vi "filter.wait.for.command.vi"(11 "filter.data in":T1 {"memory.command"."order.slot.value"."Quantity" format="%016x"; "memory.command"."order.slot.value"."OrderId" format="%016x"; "memory.command"."ticker.slot.value"."Symbol" format="%016x"; "Scratch"."OrderId" format="%016x"}) -> (2 "Ready.for.OrderBook.Command.Input":bool, 3 "filter.data out":T1 {"memory.command"."order.slot.value"."Quantity" format="%016x"; "memory.command"."order.slot.value"."OrderId" format="%016x"; "memory.command"."ticker.slot.value"."Symbol" format="%016x"; "Scratch"."OrderId" format="%016x"})   [LabVIEW 2022 SP3]
uses:
  filter.data.ctl
  filter.states.ctl
  filter.debug.ctl
  filter.debug.slot.ctl
  filter.data.scratch.ctl
  arty/orderbook/orderbook.command.ctl
  arty/orderbook/orderbook.command.type.ctl
  filter.memory.command.ctl
  ticker.slot.ctl
  order.slot.ctl
  <vilib>/rvi/Emulation/niFpgaEmulationIsFPGAContextNoSignature.vi
  <vilib>/rvi/Emulation/niFpgaSctlEmulationGetInTimedLoop.vi
  <vilib>/rvi/errors/niFpgaSetErrorForExecOnDevCompSimple.vi
  <vilib>/rvi/eio/common/nirviEmuReportErrorAndStop.vi
  <vilib>/rvi/DataTransferAndStorage/Container/Common/niFpgaContainerGetUniqueNameForEmu.vi
  <vilib>/rvi/FIFO/Fifo_Resource/nirvififoEmulationSetSize.vi
  <vilib>/rvi/FIFO/Fifo_Resource/nirviFifoEmulationQueueMgr.vi
  <instcachedir>/0/nirviFifoEmulationQueueMgr_E5CAEC123FF24DC58D834DCA3CDAA9B5.lvgen/nirviFifoEmulationQueueMgr_E5CAEC123FF24DC58D834DCA3CDAA9B5_017.vi
  <vilib>/Utility/error.llb/Clear Errors.vi
  <vilib>/rvi/FIFO/Fifo_Resource/nirvififoEmulationCreateLock.vi
  <vilib>/rvi/Emulation/niFpgaProcessEmulError.vi
  <vilib>/rvi/FIFO/Fifo_Resource/nirvififoEmulationObtainLock.vi
  <vilib>/rvi/FIFO/Fifo_Resource/nirvififoEmulationReleaseLock.vi
  <vilib>/rvi/occurrence/nirviWaitOnOccurrenceBase.vi
  <vilib>/rvi/errors/nirviReportUnexpectedCaseInternalError.vi
  <vilib>/rvi/errors/nirviReportUnexpectedCaseInternalError (U32).vi
  <vilib>/rvi/DataTransferAndStorage/Container/XNode/niFpgaContainer.xnode
  <vilib>/rvi/FIFO/Fifo_Resource/nirvififoEmulationRead.vi
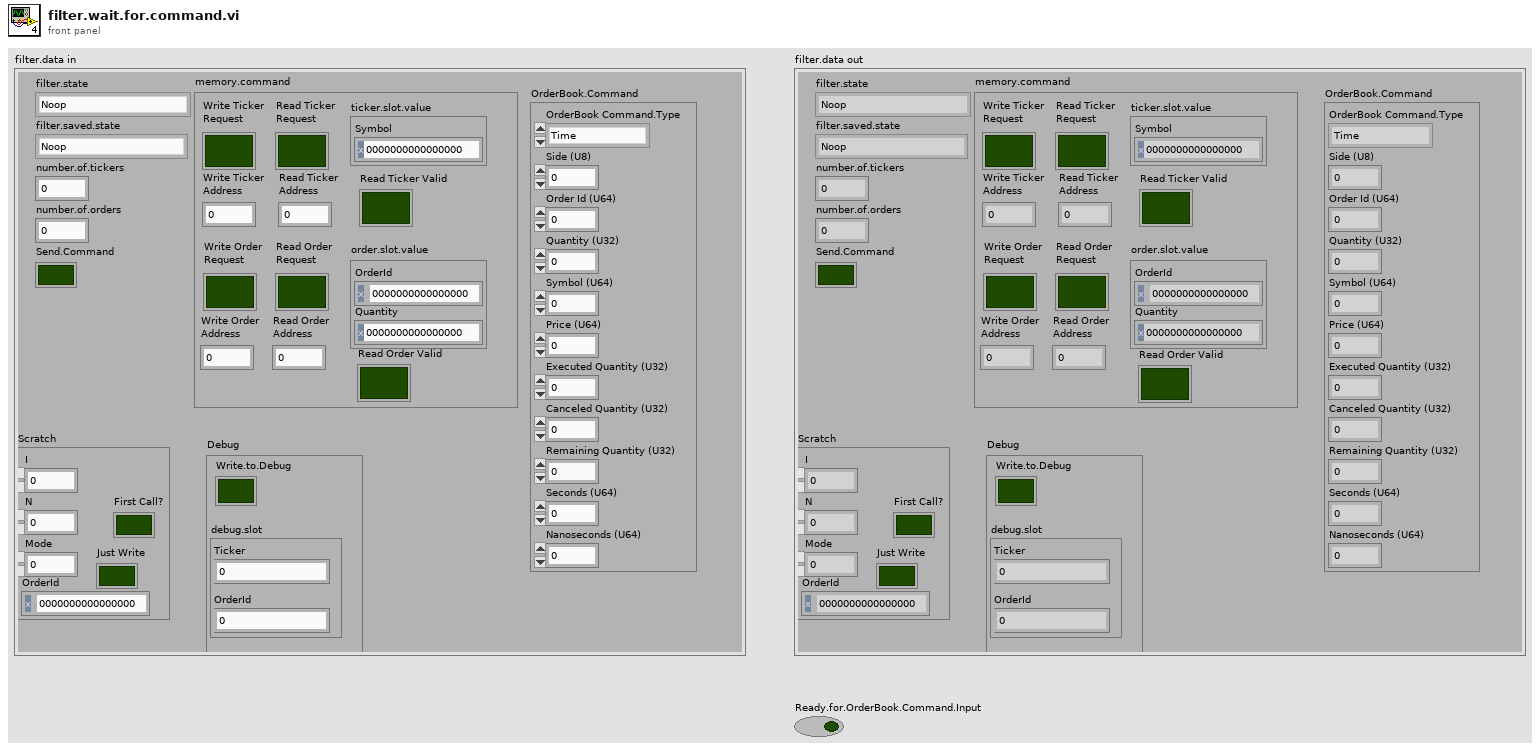
[diagram p1: front panel]
types:
  T1 = typedef "filter.data.ctl" = cluster{"filter.state":T2, "Debug":T3, "number.of.tickers":u32, "number.of.orders":u32, "filter.saved.state":T2, "Scratch":T5, "OrderBook.Command":T6, "Send.Command":bool, "memory.command":T8}
  T2 = typedef "filter.states.ctl" = enum16{"Noop", "Reset", "Debug", "Configuration", "Wait.for.Command", "Filter.Add", "Filter.Other", "Insert.Order", "Delete Order"}
  T3 = typedef "filter.debug.ctl" = cluster{"Write.to.Debug":bool, "debug.slot":T4}
  T4 = typedef "filter.debug.slot.ctl" = cluster{"Ticker":u64, "OrderId":u64}
  T5 = typedef "filter.data.scratch.ctl" = cluster{"I":u32, "N":u32, "Mode":u32, "OrderId":u64, "First Call?":bool, "Just Write":bool}
  T6 = typedef "orderbook.command.ctl" = cluster{"OrderBook Command.Type":T7, "Side (U8)":u8, "Order Id (U64)":u64, "Quantity (U32)":u32, "Symbol (U64)":u64, "Price (U64)":u64, "Executed Quantity (U32)":u32, "Canceled Quantity (U32)":u32, "Remaining Quantity (U32)":u32, "Seconds (U64)":u64, "Nanoseconds (U64)":u64}
  T7 = typedef "orderbook.command.type.ctl" = enum16{"Time", "AddOrder", "OrderExecuted", "OrderExecutedAtPrice", "ReduceSize", "ModifyOrder", "DeleteOrder", "Get.All.Orders", "Get.Top"}
  T8 = typedef "filter.memory.command.ctl" = cluster{"ticker.slot.value":T9, "order.slot.value":T10, "Write Ticker\nAddress":u32, "Write Ticker\nRequest":bool, "Read Ticker\nRequest":bool, "Read Ticker\nAddress":u32, "Read Ticker Valid":bool, "Write Order\nAddress":u32, "Write Order\nRequest":bool, "Read Order\nRequest":bool, "Read Order\nAddress":u32, "Read Order Valid":bool}
  T9 = typedef "ticker.slot.ctl" = cluster{"Symbol":u64}
  T10 = typedef "order.slot.ctl" = cluster{"OrderId":u64, "Quantity":u64}
  T11 = cluster{"OrderBook Command.Type":enum16{"Time", "AddOrder", "OrderExecuted", "OrderExecutedAtPrice", "ReduceSize", "ModifyOrder", "DeleteOrder", "Get.All.Orders", "Get.Top"}, "Side (U8)":u8, "Order Id (U64)":u64, "Quantity (U32)":u32, "Symbol (U64)":u64, "Price (U64)":u64, "Executed Quantity (U32)":u32, "Canceled Quantity (U32)":u32, "Remaining Quantity (U32)":u32, "Seconds (U64)":u64, "Nanoseconds (U64)":u64}
  T12 = enum16{"Time", "AddOrder", "OrderExecuted", "OrderExecutedAtPrice", "ReduceSize", "ModifyOrder", "DeleteOrder", "Get.All.Orders", "Get.Top"}
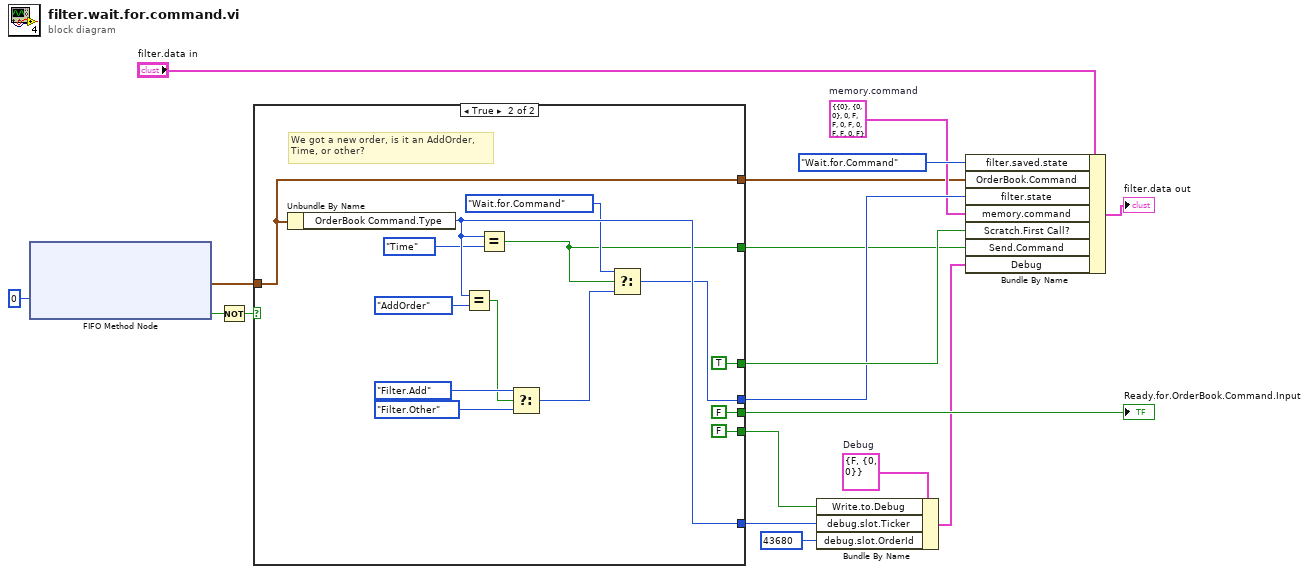
[diagram p0: block diagram]
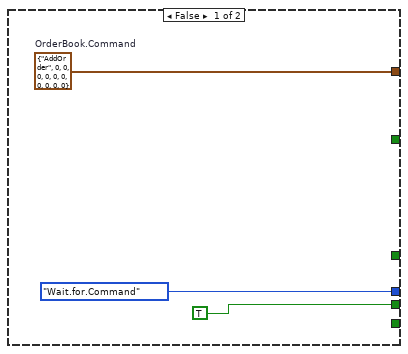
[diagram p2: hidden frame]
diagram:
  w13 = T3 {"Write.to.Debug"=FALSE, "debug.slot"={"Ticker"=0, "OrderId"=0}}  # Debug
  w12 = T8 {"ticker.slot.value"={"Symbol"=0}, "order.slot.value"={"OrderId"=0, "Quantity"=0}, "Write Ticker\nAddress"=0, "Write Ticker\nRequest"=FALSE, "Read Ticker\nRequest"=FALSE, "Read Ticker\nAddress"=0, "Read Ticker Valid"=FALSE, "Write Order\nAddress"=0, "Write Order\nRequest"=FALSE, "Read Order\nRequest"=FALSE, "Read Order\nAddress"=0, "Read Order Valid"=FALSE}  # memory.command
  n1 = xnode ("FIFO Method Node")("Timeout"=0) -> ("Element"=w8:T11, "Timed Out?"=w7:bool)  [unwired: 1 in, 1 out]
  n2 = Not(x=w7) -> (.not. x?=w9:bool)
  n3 = case shown="True" w9 {
    tunnel: w8 -> [_ w32]
    tunnel: [w19 w32] -> w10
    tunnel: [filter.states."Wait.for.Command" ("filter.state") w24] -> w16
    tunnel: [TRUE FALSE] -> w11
    tunnel: [_ FALSE] -> w17
    tunnel: [_ w27] -> w3
    tunnel: [_ TRUE ("First Call?")] -> w18
    tunnel: [_ w22] -> w1
    frame False {
      w19 = T6 {"OrderBook Command.Type"=enum."AddOrder", "Side (U8)"=0, "Order Id (U64)"=0, "Quantity (U32)"=0, "Symbol (U64)"=0, "Price (U64)"=0, "Executed Quantity (U32)"=0, "Canceled Quantity (U32)"=0, "Remaining Quantity (U32)"=0, "Seconds (U64)"=0, "Nanoseconds (U64)"=0}  # OrderBook.Command
    }
    frame True {
      # "We got a new order, is it an AddOrder,\nTime, or other?"
      n4 = Unbundle By Name(w32) -> ("OrderBook Command.Type"=w27:T12)
      n5 = Equal?(x=w27, y=T12."AddOrder") -> (x = y?=w33:bool)
      n6 = Equal?(x=w27, y=T12."Time") -> (x = y?=w22:bool)
      n7 = Select(t=filter.states."Filter.Add" ("filter.state"), s=w33, f=filter.states."Filter.Other" ("filter.state")) -> (s? t:f=w25:T2)
      n8 = Select(t=filter.states."Wait.for.Command", s=w22, f=w25) -> (s? t:f=w24:T2)
    }
  }
  "Ready.for.OrderBook.Command.Input" <- w11
  n9 = Bundle By Name(cluster=w13, "Write.to.Debug"=w17, "debug.slot.Ticker"=w3, "debug.slot.OrderId"=u64 43680 ("OrderId")) -> (w2:T3)
  n10 = Bundle By Name(cluster="filter.data in", "filter.saved.state"=filter.states."Wait.for.Command", "OrderBook.Command"=w10, "filter.state"=w16, "memory.command"=w12, "Scratch.First Call?"=w18, "Send.Command"=w1, "Debug"=w2) -> (→"filter.data out":T1)
